vi "timer.vi"() -> ()   [LabVIEW 2016]
panel:
  in  "s":bool
  out "x+y":dbl
  in  "stop":bool
  out "x-y":dbl
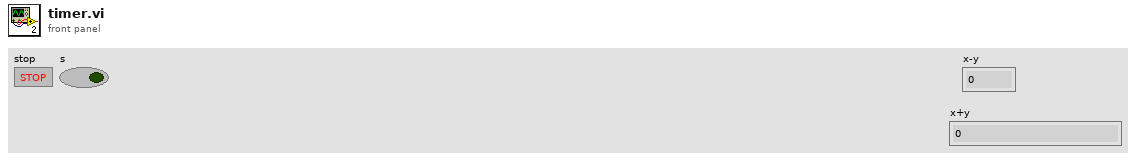
[diagram p1: front panel]
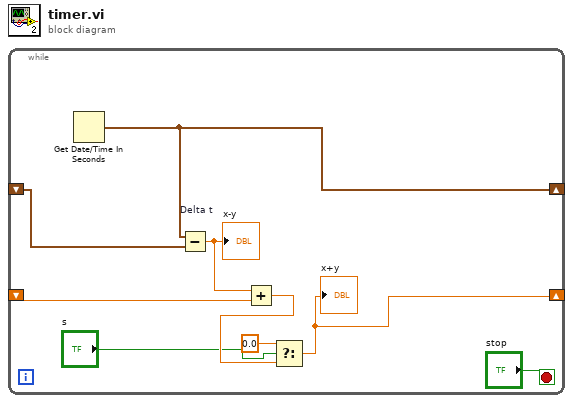
[diagram p0: block diagram]
diagram:
  n1 = while {
    shift-right: [w8] -> _
    shift-left: _ -> [w9]
    shift-right: [w2] -> _
    shift-left: _ -> [w5]
    stop <- "stop" stop-if-true
    n2 = Get Date/Time In Seconds() -> (seconds since 1Jan1904=w8:timestamp)
    n3 = Subtract "Delta t"(x=w8, y=w9) -> (x-y=w6:dbl)
    "x-y" <- w6
    n4 = Add(x=w6, y=w5) -> (x+y=w3:dbl)
    n5 = Select(t=0.0, s="s", f=w3) -> (s? t:f=w2:dbl)
    "x+y" <- w2
  }
